vi "Server.vi"() -> ()   [LabVIEW 2015]
doc: "Creates a named service and listens on the first available port. When a client connects to the service, it sends a response string to the client."
panel:
  in  "Location Y":string="You are currently accessing TCP Named Service - Server.vi from client %s on port %d."
  in  "Location X":string="You are currently accessing TCP Named Service - Server.vi from client %s on port %d."
  in  "Message Type":string="You are currently accessing TCP Named Service - Server.vi from client %s on port %d."
  in  "Stop":bool
  # "Overview: Demonstrates the use of the TCP functions to initialize a named TCP service that can send data to a client VI.\nInstructions:\n1. Run the VI.\n2. Open TCP Named Service - Client.vi and follow the instructions on its front panel.\n3. Click Stop to stop the VI."
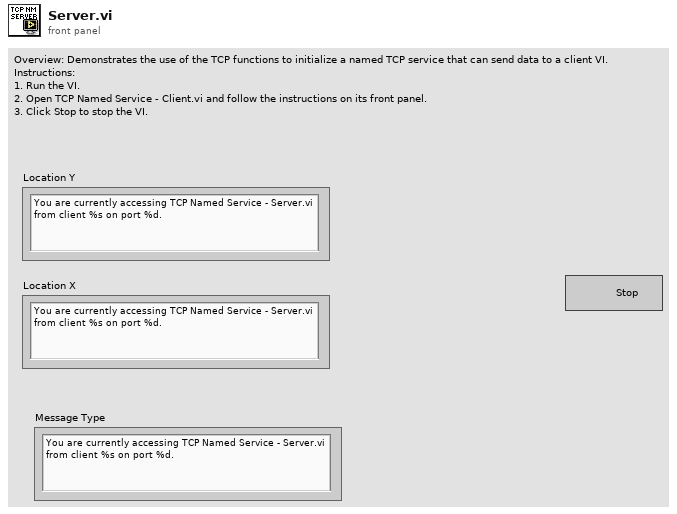
[diagram p1: front panel]
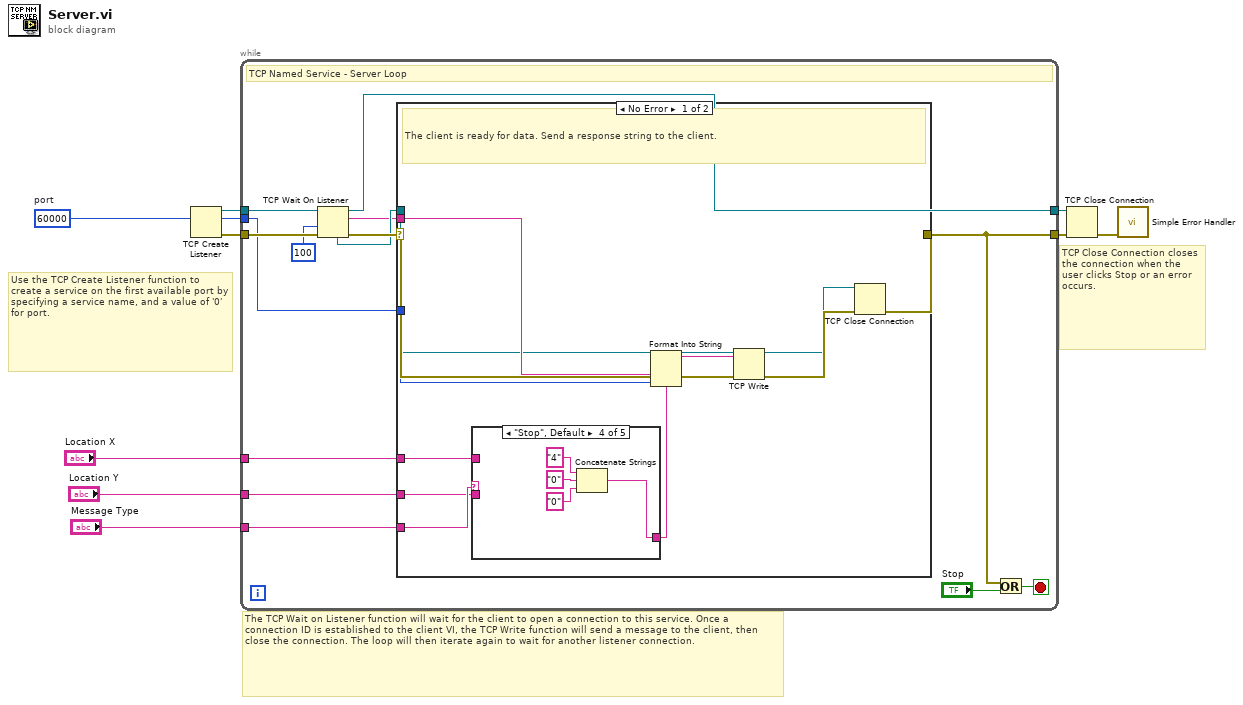
[diagram p0: block diagram]
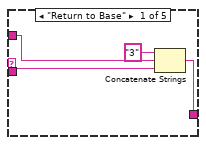
[diagram p2: hidden frame]
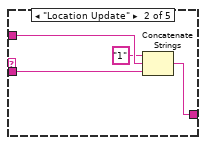
[diagram p3: hidden frame]
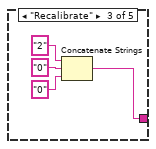
[diagram p4: hidden frame]
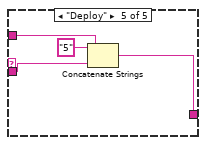
[diagram p5: hidden frame]
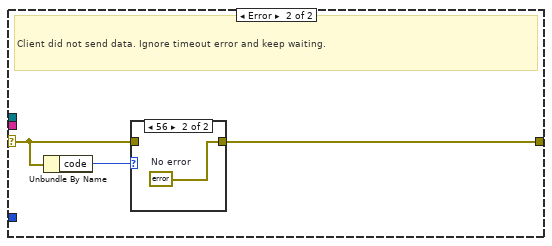
[diagram p6: hidden frame]
diagram:
  w4 = u16 60000  # port
  # "TCP Close Connection closes the connection when the user clicks Stop or an error occurs."
  # "The TCP Wait on Listener function will wait for the client to open a connection to this service. Once a connection ID is established to the client VI, the TCP Write function will send a message to the client, then close the connection. The loop will then iterate again to wait for another listener connection."
  # "Use the TCP Create Listener function to create a service on the first available port by specifying a service name, and a value of '0' for port."
  n1 = TCP Create Listener(10:w4) -> (0:w9:errorcluster, 2:w6:u16, 3:w10:refnum<k5>)  [unwired: 4 in]
  n2 = while {
    tunnel: [w17] -> w7
    tunnel: w10 -> [w24]
    tunnel: w9 -> [w22]
    tunnel: [w14] -> w8
    tunnel: w6 -> [w20]
    tunnel: "Message Type" -> [w13]
    tunnel: "Location X" -> [w12]
    tunnel: "Location Y" -> [w11]
    stop <- w19 stop-if-true
    # "TCP Named Service - Server Loop"
    n3 = TCP Wait On Listener(8:w22, 9:100 ("timeout ms (25000)"), 11:w24) -> (0:w23:errorcluster, 2:w15:string, 3:w14:refnum<k5>, 4:w21:refnum<k5>)  [unwired: 1 in, 1 out]
    n4 = case shown="No Error" w23 {
      selector: w23 -> [w36 w59]
      tunnel: [w29 w57] -> w17
      tunnel: w21 -> [w30 _]
      tunnel: w20 -> [w34 _]
      tunnel: w15 -> [w32 _]
      tunnel: w13 -> [w27 _]
      tunnel: w12 -> [w26 _]
      tunnel: w11 -> [w25 _]
      frame No Error {
        # "The client is ready for data. Send a response string to the client."
        n5 = case shown="\"Stop\", Default" w27 {
          tunnel: [w37 w41 w45 w49 w55] -> w33
          tunnel: w26 -> [w39 w44 _ _ w54]
          tunnel: w25 -> [w38 w43 _ _ w53]
          frame "Return to Base" {
            n6 = Concatenate Strings("3" ("string"), w39, w38) -> (w37:string)
          }
          frame "Location Update" {
            n7 = Concatenate Strings("1" ("string"), w44, w43) -> (w41:string)
          }
          frame "Recalibrate" {
            n8 = Concatenate Strings("2" ("string"), "0" ("string"), "0" ("string")) -> (w45:string)
          }
          frame "Stop", Default {
            n9 = Concatenate Strings("4" ("string"), "0" ("string"), "0" ("string")) -> (w49:string)
          }
          frame "Deploy" {
            n10 = Concatenate Strings("5" ("string"), w54, w53) -> (w55:string)
          }
        }
        n11 = Format Into String(format string=w33, w32, w34) -> (resulting string=w31:string)  [unwired: 2 in, 1 out]
        n12 = TCP Write(connection ID=w30, data in=w31, error in (no error)=w36) -> (connection ID out=w28:refnum<k5>, error out=w35:errorcluster)  [unwired: 1 in, 1 out]
        n13 = TCP Close Connection(connection ID=w28, error in (no error)=w35) -> (error out=w29:errorcluster)  [unwired: 1 in, 1 out]
      }
      frame Error {
        # "Client did not send data. Ignore timeout error and keep waiting."
        n14 = Unbundle By Name(w59) -> ("code"=w58:i32)
        n15 = case shown="56" w58 {
          tunnel: w59 -> [w60 _]
          tunnel: [w60 w61] -> w57
          frame Default {
          }
          frame 56 {
            w61 = errorcluster {"status"=FALSE, "code"=0, "source"=""}  # No error
          }
        }
      }
    }
    n16 = Or(x=w17, y="Stop") -> (x .or. y?=w19:bool)
  }
  n17 = TCP Close Connection(connection ID=w8, error in (no error)=w7) -> (error out=w5:errorcluster)  [unwired: 1 in, 1 out]
  n18 = call <vilib>:"Simple Error Handler.vi"("error in (no error)"=w5) -> ()  [unwired: 4 in, 5 out]
